vi "Configure Scaling Core.vi"(8 "error in (no error)":errorcluster, 9 "Scaling":dbl, 10 "AxisNumber":u8, 11 "CS++Motor in":refnum<class "CS++Motor.lvclass">) -> (0 "error out":errorcluster, 3 "CS++Motor out":refnum<class "CS++Motor.lvclass">)   [LabVIEW 2015, in "CS++Motor.lvlib" / "CS++Motor.lvclass"]
doc: "Configures the scaling from internal units (like steps) to natural units (like mm) of the axis.\n\nFor example: \"5\" means that one step corresponds to 5 times the unit."
uses:
  CS++Motor.lvclass
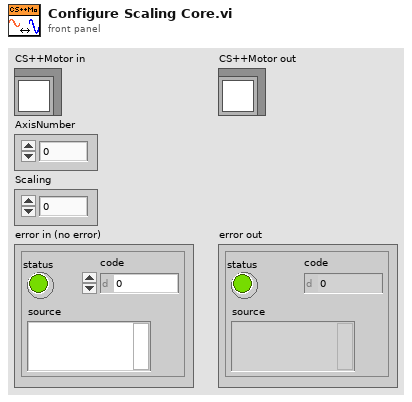
[diagram p1: front panel]
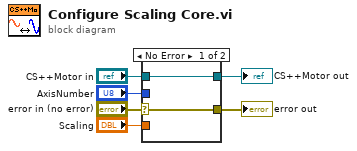
[diagram p0: block diagram]
diagram:
  n1 = case shown="No Error" "error in (no error)" {
    selector: "error in (no error)" -> [w7 w10]
    tunnel: [w7 w10] -> w5
    tunnel: [w8 w9] -> w3
    tunnel: "CS++Motor in" -> [w8 w9]
    tunnel: "AxisNumber" -> [_ _]
    tunnel: "Scaling" -> [_ _]
    frame No Error {
    }
    frame Error {
    }
  }
  "error out" <- w5
  "CS++Motor out" <- w3
